vi "Galil_firmwareDownloadFile.vi"() -> ()   [LabVIEW 2011]
panel:
  in  "Galil.IGalil":refnum<k7>
  out "Library Version:":string
  out "error out":errorcluster
  out "Connected To:":string
  in  "Connection String:":string
  # "This vi Shows how to use the firmwareDownloadFile function of the Galil Communications Library.  \n\nIf Connection String is left blank, the vi will open the connections dialog when run.  If a value is input into Connection String, the vi will attempt to connect to the controller at that address (ie COM1 19200).\n\nThe vi connects to a controller, then a file dialog box opens to choose a *.hex file.\nhex file chosen will be firmware that is downloaded to controller."
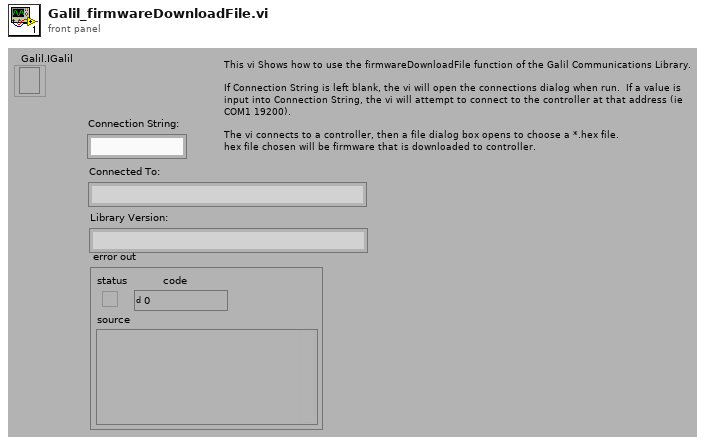
[diagram p1: front panel]
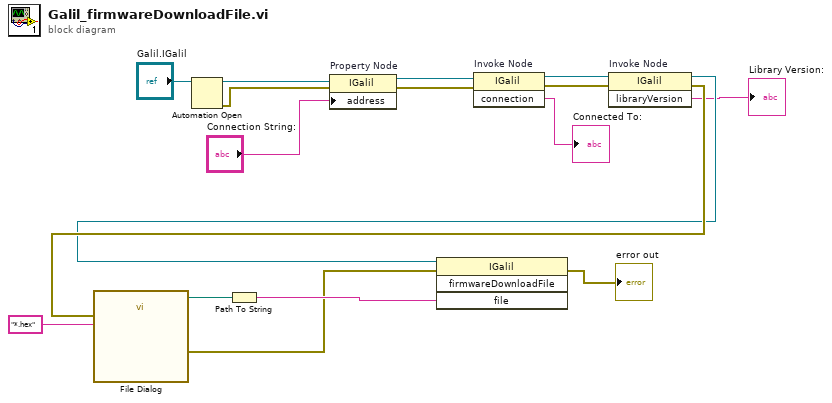
[diagram p0: block diagram]
diagram:
  n1 = Automation Open(Automation Refnum="Galil.IGalil") -> (Automation Refnum=w17:refnum<k7>, error out=w15:errorcluster)  [unwired: 1 in, 2 out]
  n2 = property on="Property Node" class="IGalil"(reference=w17, error in=w15, "address"="Connection String:") -> (reference out=w16:refnum<k7>, error out=w14:errorcluster)
  n3 = invoke on="Invoke Node" class="IGalil" method="connection"(reference=w16, error in=w14) -> (reference out=w7:refnum<k7>, error out=w6:errorcluster, "connection"=→"Connected To:":string)  [unwired: 1 in]
  n4 = invoke on="Invoke Node" class="IGalil" method="libraryVersion"(reference=w7, error in=w6) -> (reference out=w4:refnum<k7>, error out=w5:errorcluster, "libraryVersion"=→"Library Version:":string)  [unwired: 1 in]
  n5 = call "File Dialog"("error in"=w5, "pattern (all files)"="*.hex") -> ("selected path"=w11:path, "error out"=w9:errorcluster)  [unwired: 5 in, 7 out]
  n6 = Path To String(path=w11) -> (string=w10:string)
  n7 = invoke class="IGalil" method="firmwareDownloadFile"(reference=w4, error in=w9, "file"=w10) -> (error out=→"error out":errorcluster)  [unwired: 1 in, 3 out]
